vi "MGCC_FntStaMach_Interrupt_100ms.vi"() -> (2 "Boolean":bool)   [LabVIEW 2016]
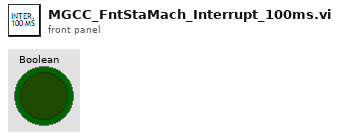
[diagram p1: front panel]
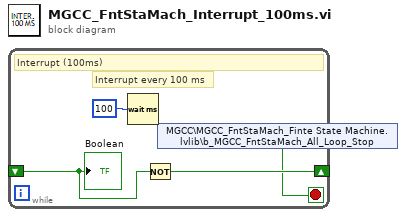
[diagram p0: block diagram]
diagram:
  n1 = while {
    shift-right: [w2] -> _
    shift-left: _ -> [w3]
    stop <- w1 stop-if-true
    # "Interrupt every 100 ms"
    # "Interrupt (100ms)"
    n2 = Wait (ms)(milliseconds to wait=u32 100) -> ()  [unwired: 1 out]
    n3 = Not(x=w3) -> (.not. x?=w2:bool)
    n4 = shared-variable "MGCC\\MGCC_FntStaMach_Finte State Machine.lvlib\\b_MGCC_FntStaMach_All_Loop_Stop"() -> (w1:bool)  [unwired: 1 in, 1 out]
    "Boolean" <- w3
  }
